vi "readTcpPacketAsString.vi"(8 "error in (no error)":errorcluster, 10 "timeout ms (1000)":i32=1000, 11 "connection ID in":refnum<k5>) -> (0 "error out":errorcluster, 2 "TcpPacket":string, 3 "connection ID out":refnum<k5>)   [LabVIEW 2018]
doc: "Read the TcpPacket as string sent by the TCP server."
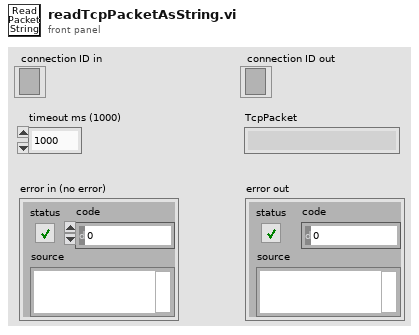
[diagram p1: front panel]
types:
  T1 = enum16{"Standard", "Buffered", "CRLF", "Immediate"}
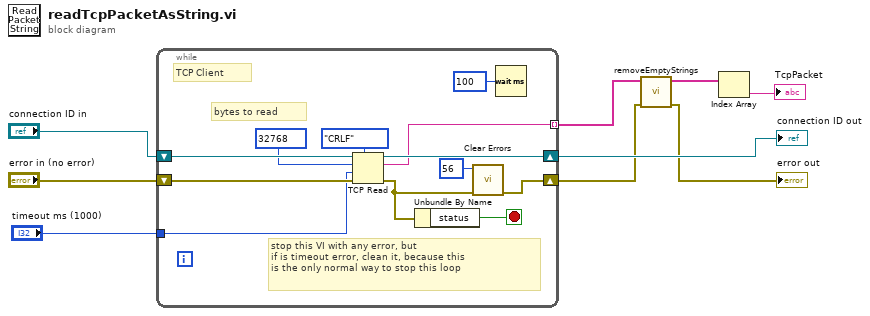
[diagram p0: block diagram]
diagram:
  n1 = while {
    shift-right: [w19] -> w9
    shift-left: "connection ID in" -> [w21]
    shift-right: [w15] -> w5
    shift-left: "error in (no error)" -> [w20]
    tunnel: [w11] -> w6 mode=indexing
    tunnel: "timeout ms (1000)" -> [w10]
    stop <- w12 stop-if-true
    # "bytes to read"
    # "stop this VI with any error, but\nif is timeout error, clean it, because this\nis the only normal way to stop this loop"
    # "TCP Client"
    n2 = TCP Read(connection ID=w21, bytes to read=32768, error in (no error)=w20, 7:T1."CRLF" ("mode (standard)"), 9:w10) -> (connection ID out=w19:refnum<k5>, data out=w11:string, error out=w13:errorcluster)
    n3 = Unbundle By Name(w13) -> ("status"=w12:bool)
    n4 = call <vilib>:"Clear Errors.vi"("error in (no error)"=w13, "specific error code to clear (0: all)"=56) -> ("error out"=w15:errorcluster)  [unwired: 4 in, 1 out]
    n5 = Wait (ms)(milliseconds to wait=u32 100) -> ()  [unwired: 1 out]
  }
  "connection ID out" <- w9
  n6 = call "removeEmptyStrings.vi"("error in (no error)"=w5, "stringArray in"=w6) -> ("error out"=→"error out":errorcluster, "stringArray out"=w3:string[])  [unwired: 8 in]
  n7 = Index Array(array=w3) -> (element=→"TcpPacket":string)  [unwired: 1 in]
